vi "Update cursors.vi"(8 "error in (no error)":errorcluster, 9 "XY Graph Reference":refnum<vi>, 10 "Diastolic IN":dbl, 11 "Systolic IN":dbl) -> (0 "error Out":errorcluster, 2 "Diastolic OUT":dbl, 3 "Systolic OUT":dbl)   [LabVIEW 2017]
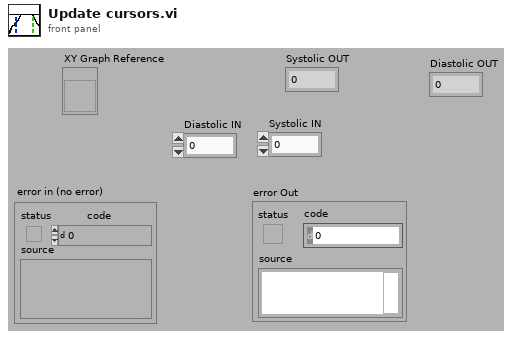
[diagram p1: front panel]
types:
  T1 = typedef "LVCursorListTypeDef.ctl" = cluster{"Name":string, "Color":u32, "Style":u8, "Point Style":u8, "Name Visible":bool, "Allow Drag":bool, "Cursor Mode":u32, "Plot":i32, "Index":i32, "Position":cluster{"X":dbl, "Y":dbl}, "X Scale":u32, "Y Scale":u32, "Watch Plots":i32[], "Watch All Plots":bool, "Plot Area":i32, "Label Offset":cluster{"X":dbl, "Y":dbl}}[]
  T2 = cluster{"Name":string, "Color":u32, "Style":u8, "Point Style":u8, "Name Visible":bool, "Allow Drag":bool, "Cursor Mode":u32, "Plot":i32, "Index":i32, "Position":cluster{"X":dbl, "Y":dbl}, "X Scale":u32, "Y Scale":u32, "Watch Plots":i32[], "Watch All Plots":bool, "Plot Area":i32, "Label Offset":cluster{"X":dbl, "Y":dbl}}
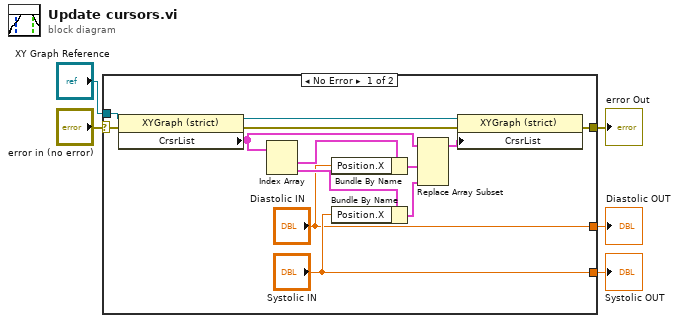
[diagram p0: block diagram]
diagram:
  n1 = case shown="No Error" "error in (no error)" {
    selector: "error in (no error)" -> [w10 w19]
    tunnel: [w6 w19] -> w4
    tunnel: ["Systolic IN" _] -> w3
    tunnel: ["Diastolic IN" _] -> w2
    tunnel: "XY Graph Reference" -> [w11 _]
    frame No Error {
      n2 = property on="Property Node" class="XYGraph (strict)"(reference=w11, error in=w10) -> (reference out=w8:refnum<vi>, error out=w7:errorcluster, "CrsrList"=w12:T1)
      n3 = Index Array(array=w12) -> (element #1=w15:T2, element #2=w16:T2)  [unwired: 2 in]
      n4 = Bundle By Name(cluster=w15, "Position.X"="Diastolic IN") -> (w17:T2)
      n5 = Bundle By Name(cluster=w16, "Position.X"="Systolic IN") -> (w18:T2)
      n6 = Replace Array Subset(array=w12, new element #1=w17, new element #2=w18) -> (w9:T1)  [unwired: 2 in]
      n7 = property on="Property Node" class="XYGraph (strict)"(reference=w8, error in=w7, "CrsrList"=w9) -> (error out=w6:errorcluster)  [unwired: 1 out]
    }
    frame Error {
    }
  }
  "error Out" <- w4
  "Systolic OUT" <- w3
  "Diastolic OUT" <- w2
